vi "NR_DeRateMatch.vi"(0 "appended path":path, 1 "deiwdata":dbl[][](array[numeric]), 2 "coded_data":dbl[][](array[numeric]), 3 "vnum":dbl, 4 "prb_num":dbl, 5 "error in (no error)":errorcluster caption="错误输入（无错误）", 6 "rvid":dbl, 7 "Qm":dbl, 8 "EN_LDPC":dbl, 10 "null_pos":dbl[][](array[numeric]), 11 "LDPC_base_graph":dbl, 12 "Zc":dbl, 14 "C":dbl, 15 "Nsym_slot":dbl, 17 "DMRS_symbol":dbl) -> (18 "dermdata":dbl[][](array[numeric]), 19 "error IO":errorcluster)   [LabVIEW 2015]
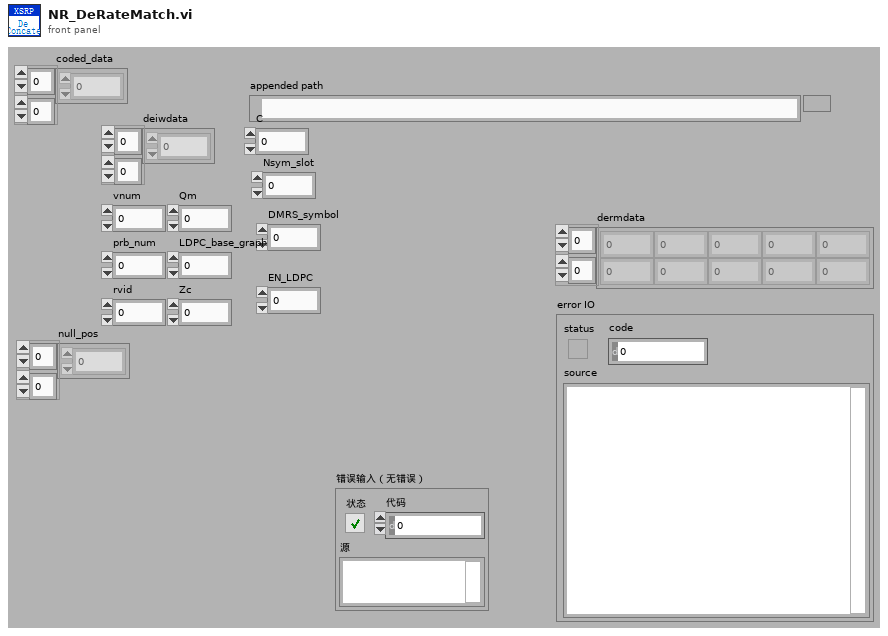
[diagram p1: front panel]
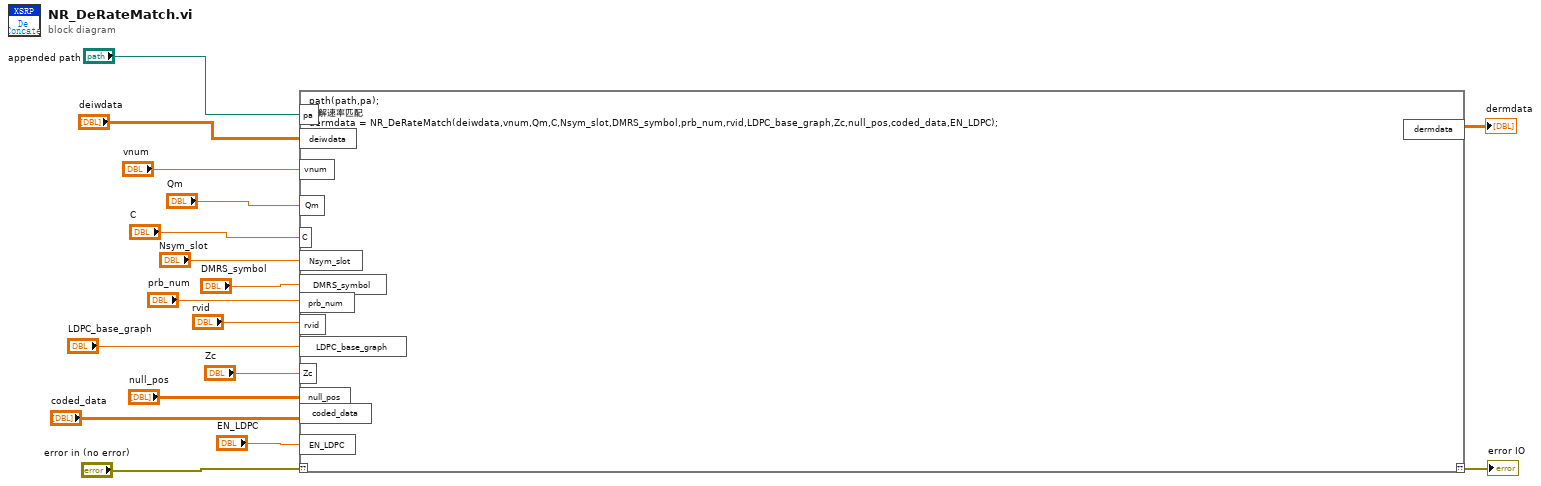
[diagram p0: block diagram]
diagram:
  n1 = script code="path(path,pa);\n%解速率匹配\ndermdata = NR_DeRateMatch(deiwdata,vnum,Qm,C,Nsym_slot,DMRS_symbol,prb_num,rvid,LDPC_base_graph,Zc,null_pos,coded_data,EN_LDPC);"("??"="error in (no error)", "pa"="appended path", "deiwdata"="deiwdata", "vnum"="vnum", "Qm"="Qm", "C"="C", "Nsym_slot"="Nsym_slot", "DMRS_symbol"="DMRS_symbol", "prb_num"="prb_num", "rvid"="rvid", "LDPC_base_graph"="LDPC_base_graph", "Zc"="Zc", "null_pos"="null_pos", "coded_data"="coded_data", "EN_LDPC"="EN_LDPC") -> ("??"=→"error IO":errorcluster, "dermdata"=→"dermdata":dbl[][])
